vi "WLAN - TV - RW - UTIL - TestVectors_11G.vi"(11 "TV_IQComposite_11G":T1={"Center Frequency(Hz)"=[2412000000.0], "OFDM Payload Length (bytes)"=0, "Standard "=0, "Array"=[], "#Avg."=0} {"Array"."OFDM Data Rate (Mbps)" items=["6", "9", "12", "18", "24", "36", "48", "54"]; "Standard" items=["80211A/G/J/P OFDM", "80211B/G DSSS", "80211G DSSSOFDM", "80211N MIMOOFDM", "80211AC MIMOOFDM"]; "Center Frequency(Hz)" format="%#_6p"}) -> (5 "new file path (Not A Path if cancelled)":path)   [LabVIEW 2011]
uses:
  <vilib>/Utility/file.llb/Write To Spreadsheet File (DBL).vi
  <vilib>/Utility/file.llb/Write To Spreadsheet File (string).vi
  Includes/WLAN - TV - RW - INC - TV_Cluster.ctl
  Includes/WLAN - TV - RW - INC - TV_IQComposite_11G.ctl
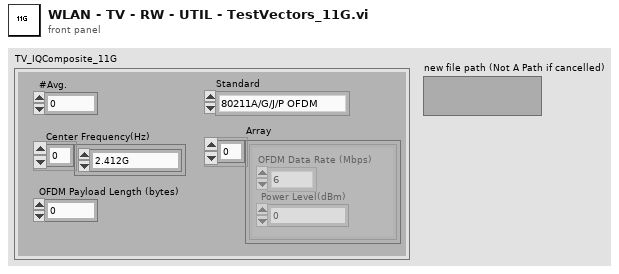
[diagram p1: front panel]
types:
  T1 = typedef "WLAN - TV - RW - INC - TV_IQComposite_11G.ctl" = cluster{"Center Frequency(Hz)":dbl[], "OFDM Payload Length (bytes)":i32, "Standard ":i32, "Array":cluster{"OFDM Data Rate (Mbps)":i32, "Power Level(dBm)":dbl}[], "#Avg.":i32}
  T2 = typedef "WLAN - TV - RW - INC - TV_Cluster.ctl" = cluster{"Standard ":string, "Channel Number":string, "Channel Frequency(Hz)":string, "Power Level(milli-dBm)":string, "Power Level(dBm)":string, "Channel Bandwidth (Hz)":string, "Idle Interval (s)":string, "OFDM Data Rate (Mbps)":string, "OFDM Payload Length (bytes)":string, "Number of Packets":string, "MCS Index":string, "Guard Interval (s)":string, "80211n PLCP Frame Format":string, "FEC Coding Type":string, "DSSS Data Rate (Mbps)":string, "DSSS Payload Length (bytes)":string, "Averages":string}
  T3 = cluster{"OFDM Data Rate (Mbps)":i32, "Power Level(dBm)":dbl}[]
  T4 = enum16{"2G Band 20M", "5G Band 20M", "5G Band 40M"}
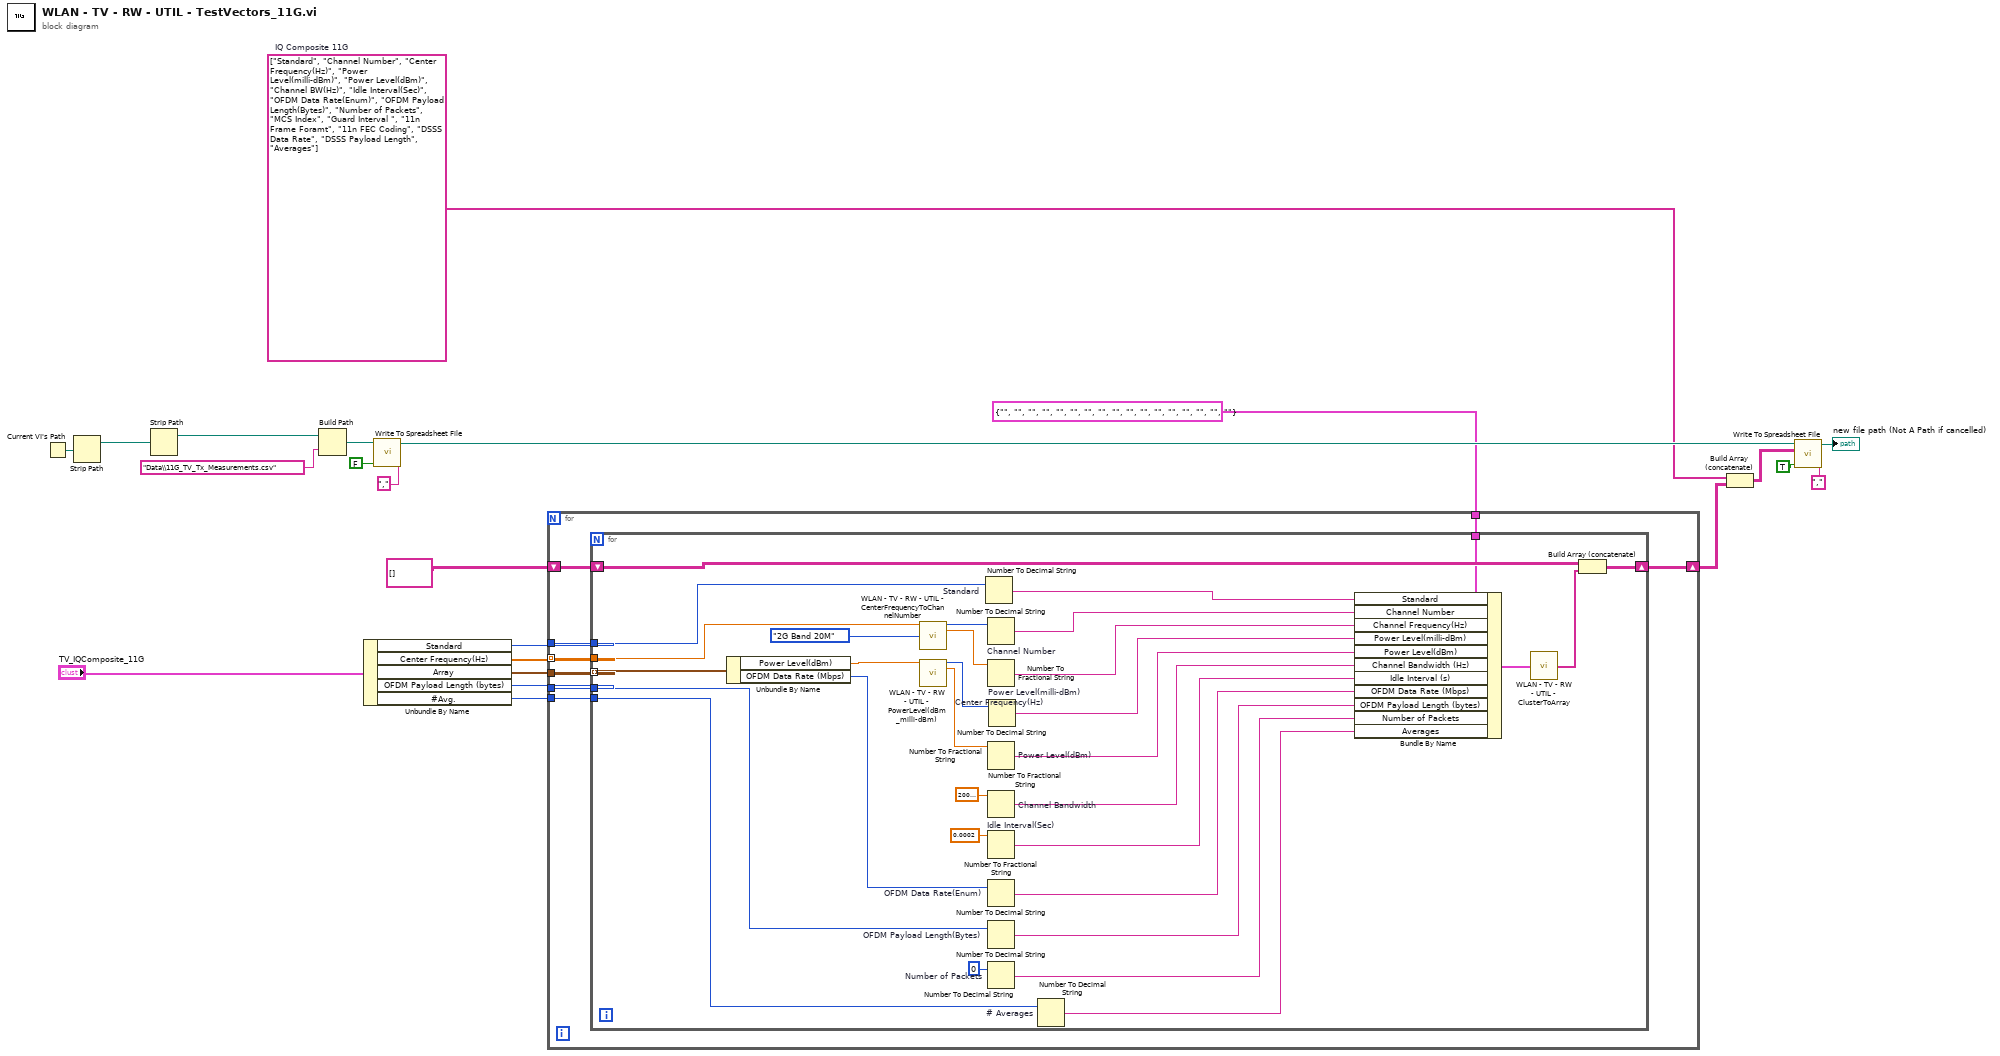
[diagram p0: block diagram]
diagram:
  w2 = string[] ["Standard", "Channel Number", "Center Frequency(Hz)", "Power Level(milli-dBm)", "Power Level(dBm)", "Channel BW(Hz)", "Idle Interval(Sec)", "OFDM Data Rate(Enum)", "OFDM Payload Length(Bytes)", "Number of Packets", "MCS Index", "Guard Interval ", "11n Frame Foramt", "11n FEC Coding", "DSSS Data Rate", "DSSS Payload Length", "Averages"]  # IQ Composite 11G
  n1 = Current VI's Path() -> (path=w21:path)
  n2 = Strip Path(path=w21) -> (stripped path=w6:path)  [unwired: 1 out]
  n3 = Strip Path(path=w6) -> (stripped path=w5:path)  [unwired: 1 out]
  n4 = Build Path(base path=w5, name or relative path="Data\\11G_TV_Tx_Measurements.csv") -> (appended path=w17:path)
  n5 = Unbundle By Name("TV_IQComposite_11G") -> ("Standard"=w9:i32, "Center Frequency(Hz)"=w15:dbl[], "Array"=w14:T3, "OFDM Payload Length (bytes)"=w13:i32, "#Avg."=w1:i32)
  n6 = call-poly <vilib>:"Write To Spreadsheet File.vi"("delimiter (\\t)"="," ("delimiter (\\t)"), "append to file? (new file:F)"=FALSE, "file path (dialog if empty)"=w17) -> ("new file path (Not A Path if cancelled)"=w16:path)  [unwired: 5 in]
  n7 = for {
    tunnel: w15 -> [w28] mode=indexing
    tunnel: w14 -> [w30]
    tunnel: w13 -> [w29]
    shift-right: [w26] -> w8
    shift-left: string[][] [] ("appended array") -> [w27]
    tunnel: w9 -> [w25]
    tunnel: T2 {"Standard "="", "Channel Number"="", "Channel Frequency(Hz)"="", "Power Level(milli-dBm)"="", "Power Level(dBm)"="", "Channel Bandwidth (Hz)"="", "Idle Interval (s)"="", "OFDM Data Rate (Mbps)"="", "OFDM Payload Length (bytes)"="", "Number of Packets"="", "MCS Index"="", "Guard Interval (s)"="", "80211n PLCP Frame Format"="", "FEC Coding Type"="", "DSSS Data Rate (Mbps)"="", "DSSS Payload Length (bytes)"="", "Averages"=""} ("TV Paramaters") -> [w24]
    tunnel: w1 -> [w23]
    n8 = for {
      tunnel: w30 -> [w60] mode=indexing
      tunnel: w29 -> [w61]
      tunnel: w28 -> [w54]
      shift-right: [w58] -> w26
      shift-left: w27 -> [w57]
      tunnel: w25 -> [w56]
      tunnel: w24 -> [w44]
      tunnel: w23 -> [w31]
      n9 = Unbundle By Name(w60) -> ("Power Level(dBm)"=w47:dbl, "OFDM Data Rate (Mbps)"=w59:i32)
      n10 = call "WLAN - TV - RW - UTIL - CenterFrequencyToChannelNumber.vi"("Center Frequency(Hz)"=w54, 7:T4."2G Band 20M" ("Frequency Band")) -> ("Coherced Channel Number"=w52:i32, "Coherced Center Frequency (Hz)"=w55:dbl)  [unwired: 12 in]
      n11 = call "WLAN - TV - RW - UTIL - PowerLevel(dBm_milli-dBm).vi"("Power Level(dBm)"=w47) -> ("Coherced Power(milli-dBm)"=w49:i32, "Coherced Power(dBm)"=w48:dbl)  [unwired: 13 in]
      n12 = Number To Decimal String "Standard"(number=w56) -> (decimal integer string=w33:string)  [unwired: 1 in]
      n13 = Number To Decimal String "Channel Number"(number=w52) -> (decimal integer string=w34:string)  [unwired: 1 in]
      n14 = Number To Fractional String "Center Frequency(Hz)"(number=w55) -> (F-format string=w35:string)  [unwired: 3 in]
      n15 = Number To Fractional String "Power Level(dBm)"(number=w48) -> (F-format string=w37:string)  [unwired: 3 in]
      n16 = Number To Fractional String "Channel Bandwidth"(number=20000000.0) -> (F-format string=w38:string)  [unwired: 3 in]
      n17 = Number To Fractional String "Idle Interval(Sec)"(number=0.0002) -> (F-format string=w39:string)  [unwired: 3 in]
      n18 = Number To Decimal String "OFDM Data Rate(Enum)"(number=w59) -> (decimal integer string=w40:string)  [unwired: 1 in]
      n19 = Number To Decimal String "OFDM Payload Length(Bytes)"(number=w61) -> (decimal integer string=w41:string)  [unwired: 1 in]
      n20 = Number To Decimal String "Number of Packets"(number=0) -> (decimal integer string=w42:string)  [unwired: 1 in]
      n21 = Number To Decimal String "Power Level(milli-dBm)"(number=w49) -> (decimal integer string=w36:string)  [unwired: 1 in]
      n22 = Number To Decimal String "# Averages"(number=w31) -> (decimal integer string=w32:string)  [unwired: 1 in]
      n23 = Bundle By Name(cluster=w44, "Standard"=w33, "Channel Number"=w34, "Channel Frequency(Hz)"=w35, "Power Level(milli-dBm)"=w36, "Power Level(dBm)"=w37, "Channel Bandwidth (Hz)"=w38, "Idle Interval (s)"=w39, "OFDM Data Rate (Mbps)"=w40, "OFDM Payload Length (bytes)"=w41, "Number of Packets"=w42, "Averages"=w32) -> (w43:T2)
      n24 = call "WLAN - TV - RW - UTIL - ClusterToArray.vi"("TV Paramaters"=w43) -> ("TV_Parameters(1-D array)"=w45:string[])  [unwired: 14 in]
      n25 = Build Array (concatenate)(w57, w45) -> (w58:string[][])
    }
  }
  n26 = Build Array (concatenate)(w2, w8) -> (w7:string[][])
  n27 = call-poly <vilib>:"Write To Spreadsheet File.vi"("delimiter (\\t)"="," ("delimiter (\\t)"), "append to file? (new file:F)"=TRUE, "2D data"=w7, "file path (dialog if empty)"=w16) -> ("new file path (Not A Path if cancelled)"=→"new file path (Not A Path if cancelled)":path)  [unwired: 4 in]
